vi "sv_Fractional-octave Analysis with IC (peak mode).vi"(0 "scaled signal [EU]":dbl[](array[numeric]) format="%.2f", 1 "peak detection mode":T1(ring), 2 "filter bank parameters":T2={"octave filter coefficients"=[{"filter structure"=enum."IIR 2nd Order", "Reverse Coefficients"=[1.0], "Forward Coefficients"=[]}], "lowpass filter coefficients"={"filter structure"=enum."IIR 2nd Order", "Reverse Coefficients"=[], "Forward Coefficients"=[]}, "number of samples to settle"=0, "number of decimation steps required"=[], "octave filter bandwidth"=[]}, 3 "internal filter state IN":T3, 4 "reset peak detection (F)":bool, 5 "filter init/cont (init:F)":bool) -> (6 "peak band power [EU^2 rms]":dbl[](array[numeric]) format="%.2f", 7 "settled?":bool, 8 "internal filter state OUT":T3)   [LabVIEW 2017, in "SoundVib_Octave_2014 standard.lvlib"]
doc: "Performs a peak fractional-octave analysis on the input signal. This VI requires the filter bank parameters and initialize filter state information the Design Octave Filter Set VI generates.\nThis VI returns the peak power in each fractional-octave band.\nThe internal filter state IN and internal filter state OUT keep track of the internal state of the filter to ensure continuous operation of the filter. To achieve this continuous operation, you must call this VI the first time with filter init/cont set to FALSE. Call it all subsequent times with filter init/cont set to TRUE. Wire the internal filter state OUT of this call to the internal filter state IN for the next call to this VI."
uses:
  <vilib>/addons/Sound and Vibration/svt_Octave/SoundVib_Octave_2014 standard.lvlib
  <vilib>/addons/_NISVFA/_Shared subVIs/Controls/svc_Octave Filter State.ctl
  <vilib>/addons/_NISVFA/_Shared subVIs/Controls/svc_Octave Filter Bank Parameters.ctl
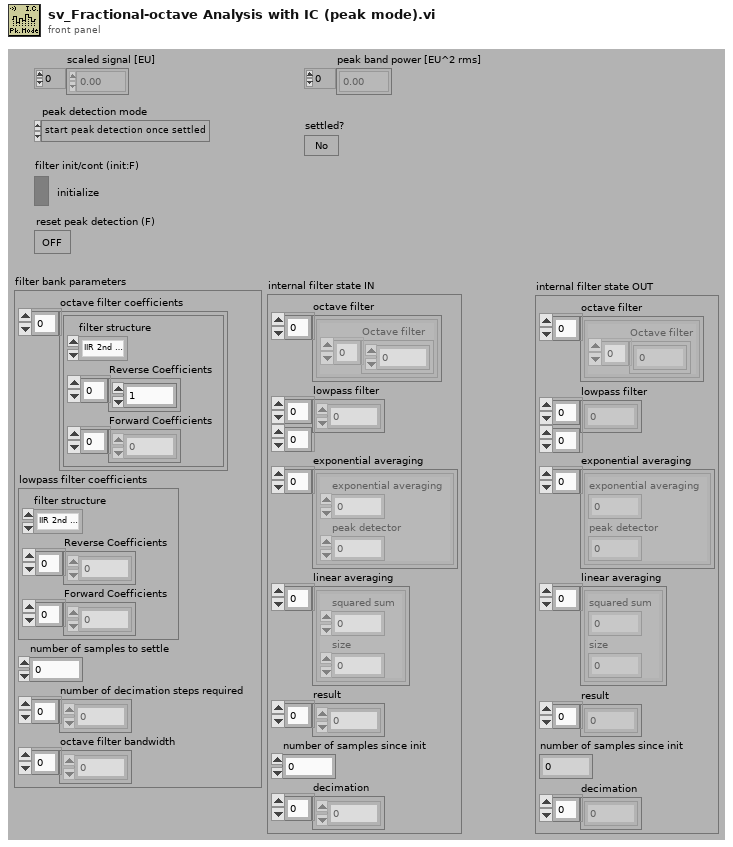
[diagram p1: front panel]
types:
  T1 = enum16{"start peak detection once settled", "continuous peak detection", "single peak detection"}
  T2 = typedef "svc_Octave Filter Bank Parameters.ctl" = cluster{"octave filter coefficients":cluster{"filter structure":enum32{"IIR 2nd Order", "IIR 4th Order"}, "Reverse Coefficients":dbl[], "Forward Coefficients":dbl[]}[], "lowpass filter coefficients":cluster{"filter structure":enum32{"IIR 2nd Order", "IIR 4th Order"}, "Reverse Coefficients":dbl[], "Forward Coefficients":dbl[]}, "number of samples to settle":u64, "number of decimation steps required":i32[], "octave filter bandwidth":dbl[]}
  T3 = typedef "svc_Octave Filter State.ctl" = cluster{"octave filter":cluster{"Octave filter":dbl[]}[], "lowpass filter":dbl[][], "exponential averaging":cluster{"exponential averaging":dbl, "peak detector":dbl}[], "linear averaging":cluster{"squared sum":dbl, "size":dbl}[], "result":dbl[], "number of samples since init":u64, "decimation":dbl[]}
  T4 = enum16{"Linear", "Exponential", "Equal confidence", "Peak"}
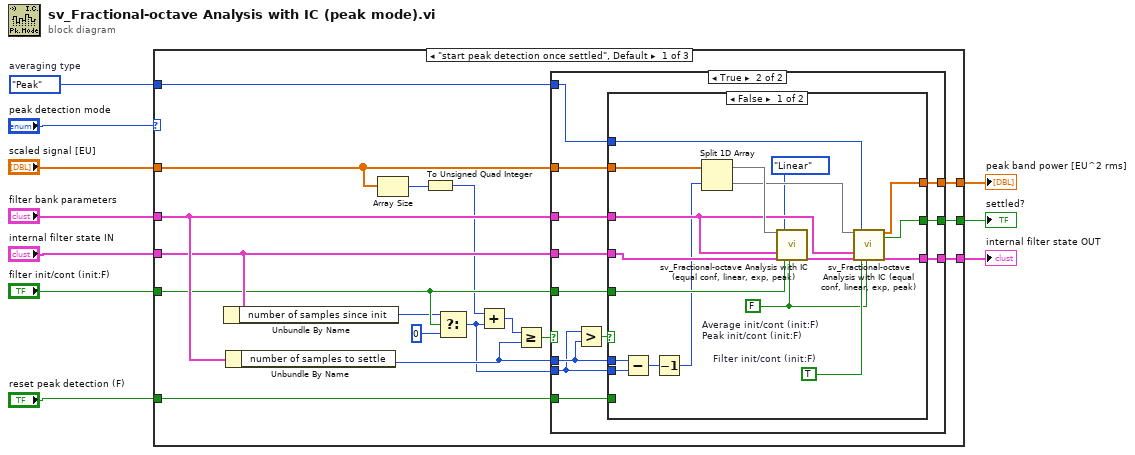
[diagram p0: block diagram]
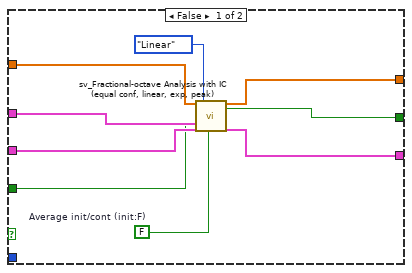
[diagram p2: hidden frame]
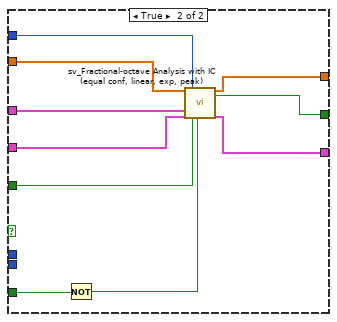
[diagram p3: hidden frame]
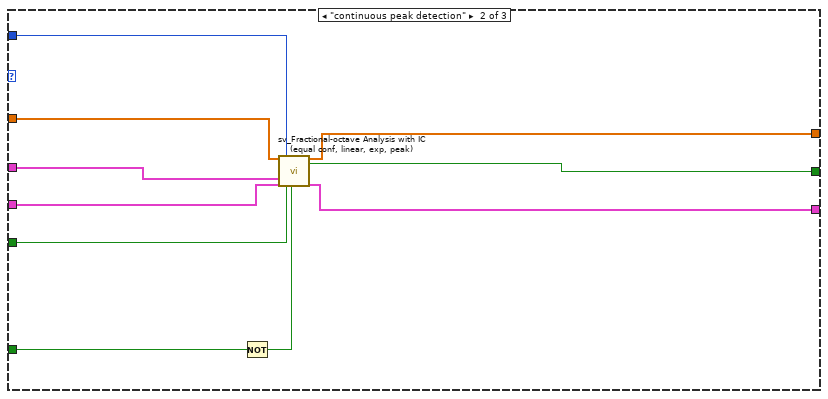
[diagram p4: hidden frame]
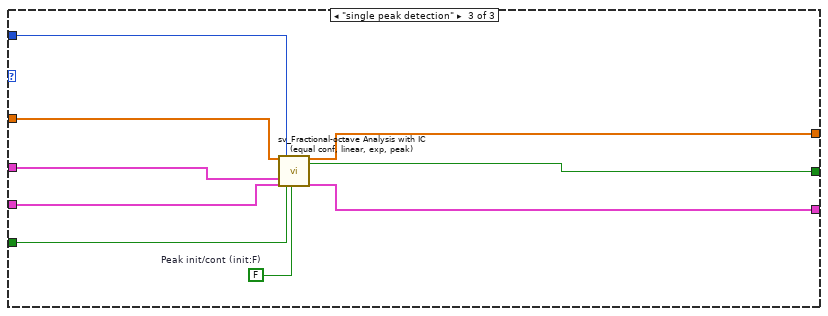
[diagram p5: hidden frame]
diagram:
  w10 = T4."Peak"  # averaging type
  n1 = case shown="\"start peak detection once settled\", Default" "peak detection mode" {
    tunnel: "scaled signal [EU]" -> [w21 w86 w95]
    tunnel: "filter bank parameters" -> [w27 w85 w94]
    tunnel: "internal filter state IN" -> [w26 w84 w93]
    tunnel: "filter init/cont (init:F)" -> [w23 w83 w92]
    tunnel: [w16 w82 w90] -> w7
    tunnel: [w15 w81 w89] -> w8
    tunnel: [w14 w80 w88] -> w9
    tunnel: "reset peak detection (F)" -> [w13 w79 _]
    tunnel: w10 -> [w11 w77 w87]
    frame "start peak detection once settled", Default {
      n2 = Unbundle By Name(w26) -> ("number of samples since init"=w22:u64)
      n3 = Unbundle By Name(w27) -> ("number of samples to settle"=w25:u64)
      n4 = Array Size(array=w21) -> (size(s)=w19:i32)
      n5 = To Unsigned Quad Integer(1:w19) -> (0:w12:u64)
      n6 = Select(t=w22, s=w23, f=u64 0) -> (s? t:f=w17:u64)
      n7 = Add(x=w12, y=w17) -> (x+y=w18:u64)
      n8 = Greater Or Equal?(x=w18, y=w25) -> (x >= y?=w24:bool)
      n9 = case shown="True" w24 {
        tunnel: w27 -> [w36 w48]
        tunnel: w21 -> [w35 w45]
        tunnel: w26 -> [w33 w47]
        tunnel: w23 -> [w32 w46]
        tunnel: w25 -> [_ w43]
        tunnel: w17 -> [_ w42]
        tunnel: [w31 w41] -> w16
        tunnel: [w30 w40] -> w15
        tunnel: [w29 w39] -> w14
        tunnel: w13 -> [_ w38]
        tunnel: w11 -> [_ w37]
        frame False {
          w34 = FALSE  # Average init/cont (init:F)
          n10 = call <vilib>:"sv_Fractional-octave Analysis with IC (equal conf, linear, exp, peak).vi"("scaled signal [EU]"=w35, "filter bank parameters"=w36, "internal filter state IN"=w33, "averaging type"=T4."Linear", "filter init/cont (init:F)"=w32, "average init/cont (cont:T)"=w34) -> ("band power [EU^2 rms]"=w31:dbl[], "settled?"=w30:bool, "internal filter state OUT"=w29:T3)  [unwired: 9 in, 2 out]
        }
        frame True {
          n11 = Greater?(x=w42, y=w43) -> (0:w44:bool)
          n12 = case shown="False" w44 {
            tunnel: w48 -> [w56 w76]
            tunnel: w47 -> [w61 w75]
            tunnel: w46 -> [w60 w74]
            tunnel: w45 -> [w66 w73]
            tunnel: w43 -> [w65 _]
            tunnel: w42 -> [w64 _]
            tunnel: [w54 w72] -> w41
            tunnel: [w53 w71] -> w40
            tunnel: [w52 w70] -> w39
            tunnel: w38 -> [_ w69]
            tunnel: w37 -> [w50 w67]
            frame False {
              w59 = TRUE  # Filter init/cont (init:F)
              w55 = FALSE  # Average init/cont (init:F) Peak init/cont (init:F)
              n13 = Subtract(x=w65, y=w64) -> (x-y=w63:u64)
              n14 = Decrement(x=w63) -> (x-1=w51:u64)
              n15 = Split 1D Array(array=w66, index=w51) -> (first subarray=w62:dbl[], second subarray=w58:dbl[])
              n16 = call <vilib>:"sv_Fractional-octave Analysis with IC (equal conf, linear, exp, peak).vi"("scaled signal [EU]"=w62, "filter bank parameters"=w56, "internal filter state IN"=w61, "averaging type"=T4."Linear", "filter init/cont (init:F)"=w60, "average init/cont (cont:T)"=w55) -> ("internal filter state OUT"=w57:T3)  [unwired: 9 in, 4 out]
              n17 = call <vilib>:"sv_Fractional-octave Analysis with IC (equal conf, linear, exp, peak).vi"("scaled signal [EU]"=w58, "filter bank parameters"=w56, "internal filter state IN"=w57, "averaging type"=w50, "filter init/cont (init:F)"=w59, "average init/cont (cont:T)"=w55) -> ("band power [EU^2 rms]"=w54:dbl[], "settled?"=w53:bool, "internal filter state OUT"=w52:T3)  [unwired: 9 in, 2 out]
            }
            frame True {
              n18 = Not(x=w69) -> (.not. x?=w68:bool)
              n19 = call <vilib>:"sv_Fractional-octave Analysis with IC (equal conf, linear, exp, peak).vi"("scaled signal [EU]"=w73, "filter bank parameters"=w76, "internal filter state IN"=w75, "averaging type"=w67, "filter init/cont (init:F)"=w74, "average init/cont (cont:T)"=w68) -> ("band power [EU^2 rms]"=w72:dbl[], "settled?"=w71:bool, "internal filter state OUT"=w70:T3)  [unwired: 9 in, 2 out]
            }
          }
        }
      }
    }
    frame "continuous peak detection" {
      n20 = Not(x=w79) -> (.not. x?=w78:bool)
      n21 = call <vilib>:"sv_Fractional-octave Analysis with IC (equal conf, linear, exp, peak).vi"("scaled signal [EU]"=w86, "filter bank parameters"=w85, "internal filter state IN"=w84, "averaging type"=w77, "filter init/cont (init:F)"=w83, "average init/cont (cont:T)"=w78) -> ("band power [EU^2 rms]"=w82:dbl[], "settled?"=w81:bool, "internal filter state OUT"=w80:T3)  [unwired: 9 in, 2 out]
    }
    frame "single peak detection" {
      w91 = FALSE  # Peak init/cont (init:F)
      n22 = call <vilib>:"sv_Fractional-octave Analysis with IC (equal conf, linear, exp, peak).vi"("scaled signal [EU]"=w95, "filter bank parameters"=w94, "internal filter state IN"=w93, "averaging type"=w87, "filter init/cont (init:F)"=w92, "average init/cont (cont:T)"=w91) -> ("band power [EU^2 rms]"=w90:dbl[], "settled?"=w89:bool, "internal filter state OUT"=w88:T3)  [unwired: 9 in, 2 out]
    }
  }
  "peak band power [EU^2 rms]" <- w7
  "internal filter state OUT" <- w9
  "settled?" <- w8
